vi "Get Input Channel Group.vi"(8 "error in":errorcluster, 10 "Group Name":string, 11 "ChannelRefs":T2) -> (0 "error out":errorcluster, 2 "Channel Group":T1, 3 "ChannelRefs":T2)   [LabVIEW 2026, in "Template.lvlib" / "Template.lvclass"]
uses:
  Template.lvclass
  Template.lvclass/Template.ctl
panel:
  out "found?":bool
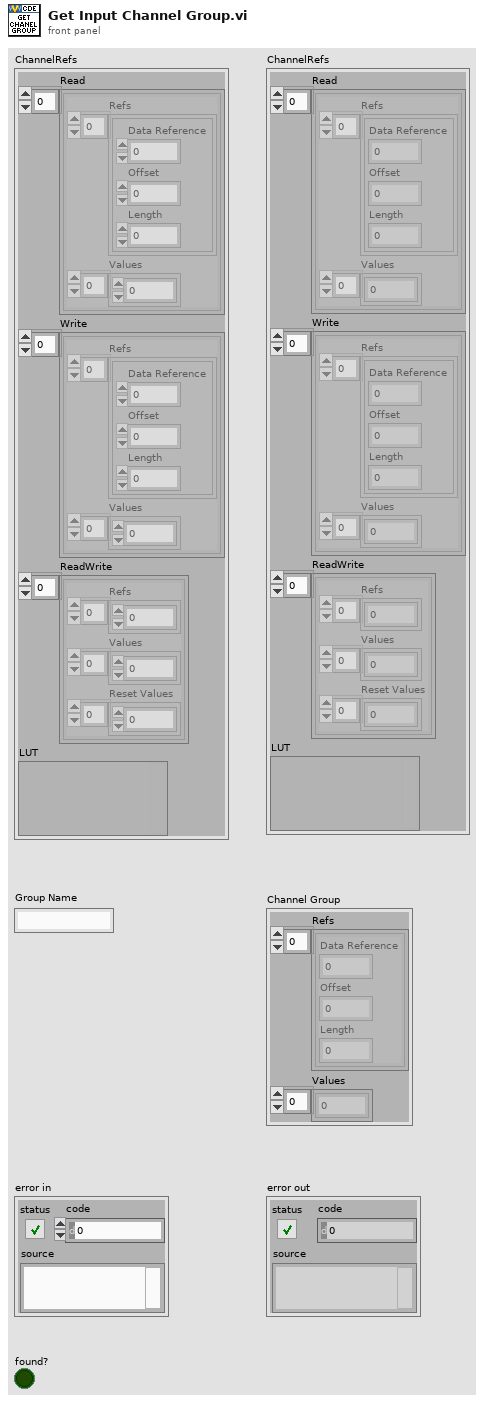
[diagram p1: front panel]
types:
  T1 = cluster{"Refs":cluster{"Data Reference":i32, "Offset":u64, "Length":u64}[], "Values":dbl[]}
  T2 = cluster{"Read":cluster{"Refs":cluster{"Data Reference":i32, "Offset":u64, "Length":u64}[], "Values":dbl[]}[], "Write":cluster{"Refs":cluster{"Data Reference":i32, "Offset":u64, "Length":u64}[], "Values":dbl[]}[], "ReadWrite":cluster{"Refs":i32[], "Values":dbl[], "Reset Values":dbl[]}[], "LUT":variant}
  T3 = enum16{"Output/Write", "Input/Read", "Input/ReadWrite"}
  T4 = cluster{"Refs":cluster{"Data Reference":i32, "Offset":u64, "Length":u64}[], "Values":dbl[]}[]
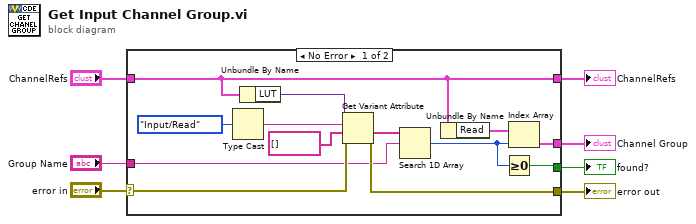
[diagram p0: block diagram]
diagram:
  n1 = case shown="No Error" "error in" {
    selector: "error in" -> [w20 w22]
    tunnel: [w19 w22] -> w6
    tunnel: [w18 _] -> w5
    tunnel: "Group Name" -> [w16 _]
    tunnel: [w10 _] -> w3
    tunnel: "ChannelRefs" -> [w11 w21]
    tunnel: [w11 w21] -> w1
    frame No Error {
      n2 = Type Cast(x=T3."Input/Read" ("Type")) -> (*(type *) &x=w12:string)  [unwired: 1 in]
      n3 = Unbundle By Name(w11) -> ("LUT"=w13:variant)
      n4 = Get Variant Attribute(Variant=w13, name=w12, default value (empty Variant)=string[] [], error in=w20) -> (value=w17:string[], error out=w19:errorcluster)  [unwired: 2 out]
      n5 = Search 1D Array(1D array=w17, element=w16) -> (index of element=w14:i32)  [unwired: 1 in]
      n6 = Unbundle By Name(w11) -> ("Read"=w9:T4)
      n7 = Greater Or Equal To 0?(x=w14) -> (x >= 0?=w10:bool)
      n8 = Index Array(array=w9, index=w14) -> (element=w18:T1)
    }
    frame Error {
    }
  }
  "ChannelRefs" <- w1
  "found?" <- w3
  "Channel Group" <- w5
  "error out" <- w6
